vi "Make DLL Param(Read Profile Rsp).vi"(1 "Read Profile Rsp":T2) -> (0 "pRsp":T1)   [LabVIEW 2014, in "Keyence LJ-V7000.lvlib"]
uses:
  Keyence LJ-V7000.lvlib
  Public/Clusters/Read Profile Rsp.ctl
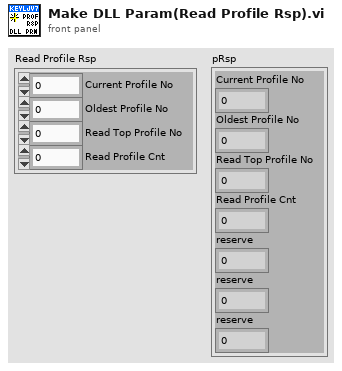
[diagram p1: front panel]
types:
  T1 = cluster{"Current Profile No":u32, "Oldest Profile No":u32, "Read Top Profile No":u32, "Read Profile Cnt":u8, "reserve":u8, "reserve":u8, "reserve":u8}
  T2 = typedef "Keyence LJ-V7000.lvlib/Read Profile Rsp.ctl" = cluster{"Current Profile No":u32, "Oldest Profile No":u32, "Read Top Profile No":u32, "Read Profile Cnt":u8}
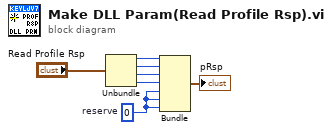
[diagram p0: block diagram]
diagram:
  w2 = u8 0  # reserve
  n1 = Unbundle("Read Profile Rsp") -> ("Current Profile No"=w6:u32, "Oldest Profile No"=w5:u32, "Read Top Profile No"=w4:u32, "Read Profile Cnt"=w3:u8)
  n2 = Bundle("Current Profile No"=w6, "Oldest Profile No"=w5, "Read Top Profile No"=w4, "Read Profile Cnt"=w3, "reserve"=w2, "reserve"=w2, "reserve"=w2) -> (→"pRsp":T1)  [unwired: 1 in]
